vi "Read Cycle.vi"(8 "error in (no error)":errorcluster, 11 "Change Speaker Switch State in":refnum<class "Change Speaker Switch State.lvclass">) -> (0 "error out":errorcluster, 2 "Cycle":bool, 3 "Change Speaker Switch State out":refnum<class "Change Speaker Switch State.lvclass">)   [LabVIEW 2014, in "ePAS Library.lvlib" / "Change Speaker Switch State.lvclass"]
uses:
  Change Speaker Switch State.lvclass
  Change Speaker Switch State.lvclass/Change Speaker Switch State.ctl
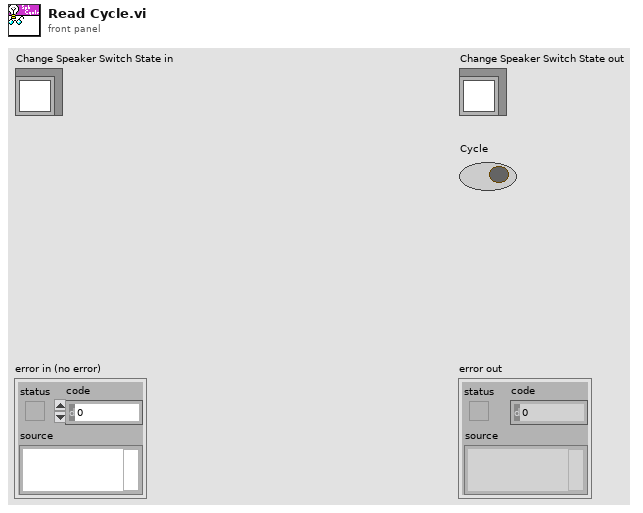
[diagram p1: front panel]
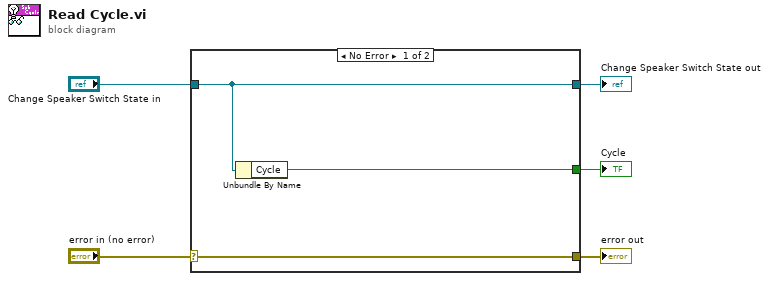
[diagram p0: block diagram]
diagram:
  n1 = case shown="No Error" "error in (no error)" {
    selector: "error in (no error)" -> [w8 w9]
    tunnel: [w8 w9] -> w4
    tunnel: [w7 w10] -> w2
    tunnel: "Change Speaker Switch State in" -> [w7 w10]
    tunnel: [w6 _] -> w1
    frame No Error {
      n2 = Unbundle By Name(w7) -> ("Cycle"=w6:bool)
    }
    frame Error {
    }
  }
  "error out" <- w4
  "Change Speaker Switch State out" <- w2
  "Cycle" <- w1
